vi "Clone.vi"(0 "image in":refnum<class "MSC Image.lvclass">, 5 "error in (no error)":errorcluster) -> (14 "image out":refnum<class "MSC Image.lvclass">, 15 "clone image out":refnum<class "MSC Image.lvclass">, 19 "error out":errorcluster)   [LabVIEW 2014, in "MSC Image.lvclass"]
doc: "This vi copies all elements from the image into a new object.\nIt is necessary to delete both references to prevent memory leaks."
uses:
  MSC Image.lvclass
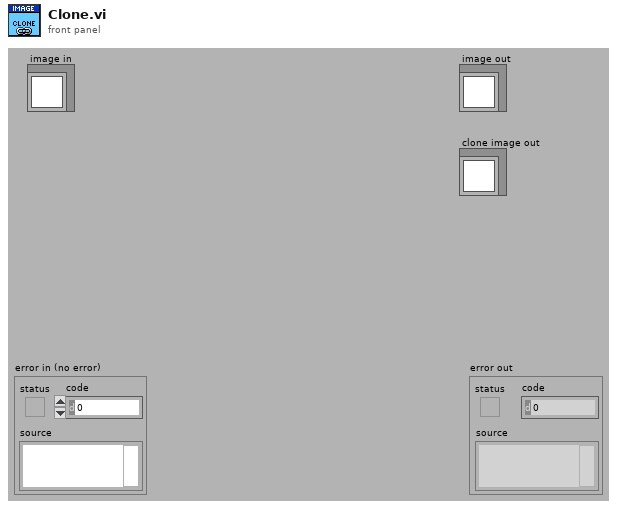
[diagram p1: front panel]
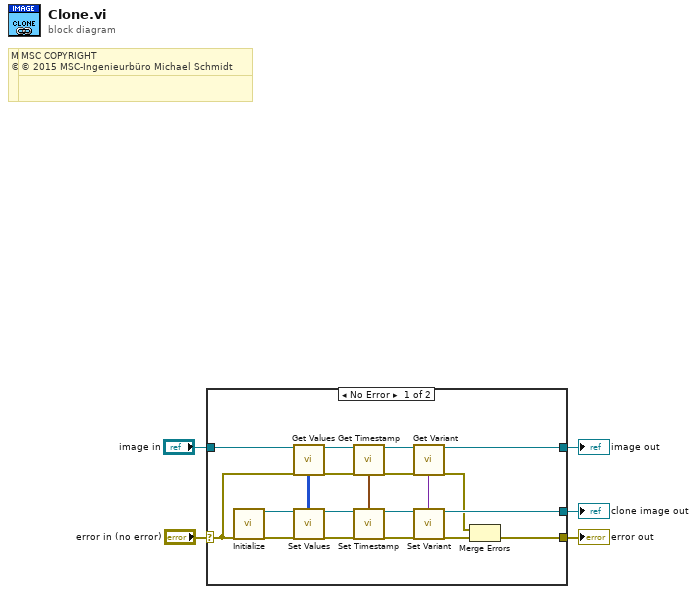
[diagram p0: block diagram]
diagram:
  # "MSC COPYRIGHT\n© 2016 MSC-Ingenieurbüro Michael Schmidt"
  # "MSC COPYRIGHT\n© 2016 MSC-Ingenieurbüro Michael Schmidt"
  # "MSC COPYRIGHT\n© 2015 MSC-Ingenieurbüro Michael Schmidt"
  # "MSC COPYRIGHT\n© 2015 MSC-Ingenieurbüro Michael Schmidt"
  n1 = case shown="No Error" "error in (no error)" {
    selector: "error in (no error)" -> [w6 w31]
    tunnel: [w7 w31] -> w4
    tunnel: [w21 w30] -> w2
    tunnel: "image in" -> [w29 w30]
    tunnel: [w20 _] -> w1
    frame No Error {
      n2 = call "Initialize.vi"("error in (no error)"=w6) -> ("image out"=w28:refnum<class "MSC Image.lvclass">, "error out"=w19:errorcluster)  [unwired: 17 in]
      n3 = call-dynamic "Get Values.vi"("image in"=w29, "error in (no error)"=w6) -> ("imageData BGR"=w12:u32[][], "image out"=w23:refnum<class "MSC Image.lvclass">, "imageData U8"=w16:u8[][], "imageData U16"=w15:u16[][], "imageData Single"=w14:sgl[][], "imageData Double"=w13:dbl[][], "error out"=w25:errorcluster)  [unwired: 10 in, 1 out]
      n4 = call-dynamic "Set Values.vi"("image in"=w28, "imageData U8"=w16, "imageData U16"=w15, "imageData Single"=w14, "imageData Double"=w13, "error in (no error)"=w19, "imageData BGR"=w12) -> ("image out"=w27:refnum<class "MSC Image.lvclass">, "error out"=w18:errorcluster)  [unwired: 11 in]
      n5 = call-dynamic "Get Timestamp.vi"("image in"=w23, "error in (no error)"=w25) -> ("image out"=w22:refnum<class "MSC Image.lvclass">, "Time Stamp"=w11:timestamp, "error out"=w24:errorcluster)  [unwired: 15 in]
      n6 = call-dynamic "Set Timestamp.vi"("image in"=w27, "Time Stamp"=w11, "error in (no error)"=w18) -> ("image out"=w26:refnum<class "MSC Image.lvclass">, "error out"=w17:errorcluster)  [unwired: 15 in]
      n7 = call-dynamic "Get Variant.vi"("image in"=w22, "error in (no error)"=w24) -> ("image out"=w21:refnum<class "MSC Image.lvclass">, "Variant"=w10:variant, "error out"=w8:errorcluster)  [unwired: 15 in]
      n8 = call-dynamic "Set Variant.vi"("image in"=w26, "Variant"=w10, "error in (no error)"=w17) -> ("image out"=w20:refnum<class "MSC Image.lvclass">, "error out"=w9:errorcluster)  [unwired: 15 in]
      n9 = Merge Errors(w8, w9) -> (w7:errorcluster)
    }
    frame Error {
    }
  }
  "error out" <- w4
  "image out" <- w2
  "clone image out" <- w1
